vi "IV_Sweep_program1_CEM_Mod2.vi"() -> ()   [LabVIEW 2013]
doc: "I. Description:\nThis example demonstrates how to continuously acquire and generate data at the same time, synchronized with one another.\n\nII. Instructions for Running:\n1. Select the physical channel to correspond to where your signal is input on the DAQ device. Also, select the corresponding channel for where your signal is being generated.\n2. Enter the minimum and maximum voltage ranges.\nNote: For better accuracy try to match the input range to the expected voltage level of the measured signal.\n3. Set the sample rate of the acquisition.\nNote: The rate should be at least twice as fast as the maximum frequency component of the signal being acquired. \n6. Select the Rate for the generation\n7. Select what type of signal to generate and the amplitude.\nNote: This example requires two DMA channels to run. If your hardware does not support two DMA channels, you need to set the Data Transfer Mechanism property for the Analog Output Task to use \"Interrupts\". The Data Transfer Mechanism property is located in the DAQmx Channel Property hierarchy at:\n\nDAQmx Channel Property Node>>Analog Output>>General Properties>>Advanced>>Data Transfer and Memory>>Data Transfer Mechanism\n\nRefer to your device documentation to determine how many DMA channels are supported for your hardware.\n\nIII. Block Diagram Steps:\n1. Create an analog input voltage channel. Also, create an analog output voltage channel.\n2. Set the rate for the sample clock. Additionally, define the sample mode to be continuous. Also, set the sample clock rate for the signal generation.\n2a. Call the Get Terminal Name with Device Prefix VI. This will take a Task and a terminal and create a properly formatted device + terminal name to use as the source of the Trigger.\n3. Define the parameters for a Digital Edge Start Trigger. Set the Analog output to trigger off the AI Start Trigger. This is an internal trigger signal.\n4. Use the Basic Function Generator VI to create the signal to be generated.\n5. Call the Start VI to arm the two functions. Make sure the analog output is armed before the analog input. This will ensure both will start at the same time.\n6. Read the waveform data in a loop until the user hits the stop button or an error occurs. The Is Task Done? VI is used to check for errors in the Analog Output Task.\n7. Call the Clear VI to Clear the Task\n8. Use the popup dialog box to display an error if any.\n\nIV. I/O Connections Overview:\nMake sure your signal input/output terminals match the Physical Channel I/O controls."
uses:
  <vilib>/Utility/error.llb/DialogType.ctl
  <vilib>/DAQmx/read.llb/DAQmx Read (Analog 1D DBL NChan 1Samp).vi
  <vilib>/DAQmx/write.llb/DAQmx Write (Analog DBL 1Chan 1Samp).vi
  <vilib>/DAQmx/create/channels.llb/DAQmx Create Channel (AO-Voltage-Basic).vi
  <vilib>/DAQmx/create/channels.llb/DAQmx Create Channel (AI-Voltage-Basic).vi
  <vilib>/DAQmx/configure/timing.llb/DAQmx Timing (Sample Clock).vi
  <vilib>/DAQmx/miscellaneous.llb/DAQmx Fill In Error Info.vi
  <vilib>/Utility/file.llb/Write To Spreadsheet File (DBL).vi
  <vilib>/Utility/file.llb/Write To Spreadsheet File (I64).vi
panel:
  out "Numeric":i32
  out "x/y":dbl
  in  "Sweep Amplitude":dbl=1.0
  in  "Stop Sweep":bool
  out "Connections 2":string="AI0=Current\nAI1=Bias\nAI2=dI/dV\nAI3=d2I/dV2\nAI4=X-Axis\nAI5=Z-Axis\n"
  out "Connections":string="AO0=Bias\nAO1=Z-axis\nAO2=X-Axis\nAO3=NA"
  in  "Columns":string
  out "Save Indicator":bool
  in  "Update Bias":bool
  in  "Save IV":bool
  in  "Save Decay":bool
  in  "Sweep Bias":bool
  in  "Step Z":bool
  in  "Comment":string="Molecule=C8\nGain=10nA\nBias Gain=div/1\nSweep Freq.=0.005Hz\nRef. Bias=5mV\nRef. Freq=4.33kHz\nGain LIA1=0.5mV\nTC LIA1=300ms\nGain LIA2=\nTC LIA2=\nLIA1=EGG"
  in  "Number Recorded":i32
  in  "DATA Filename":string="Data_"
  in  "Data Directory":path=path "E:/Research/Data"
  out "d2I/dV2":cluster{dbl[], dbl[]}(graph)
  out "dI/dV":cluster{dbl[], dbl[]}(graph)
  out "IV":cluster{dbl[], dbl[]}(graph)
  in  "# Samples":i32=2000
  in  "Frequency (Hz)":dbl=1.0
  in  "stop 3":bool
  in  "Bias":dbl caption="Bias Start Point" step=0.1 format="%_3g"
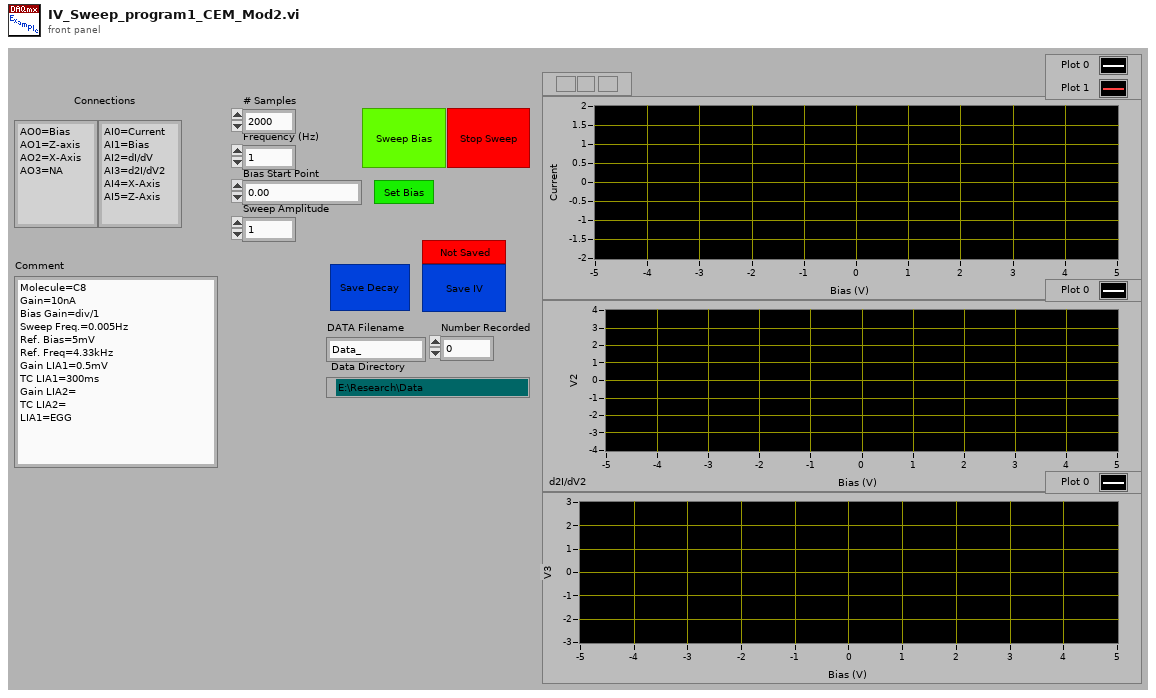
[diagram p1: front panel]
types:
  T1 = enum16{"open", "replace", "create", "open or create", "replace or create", "replace or create with confirmation"}
  T2 = typedef "DialogType.ctl" = u16
  T3 = cluster{dbl[], dbl[], dbl[], dbl[], dbl[], dbl[], dbl[]}
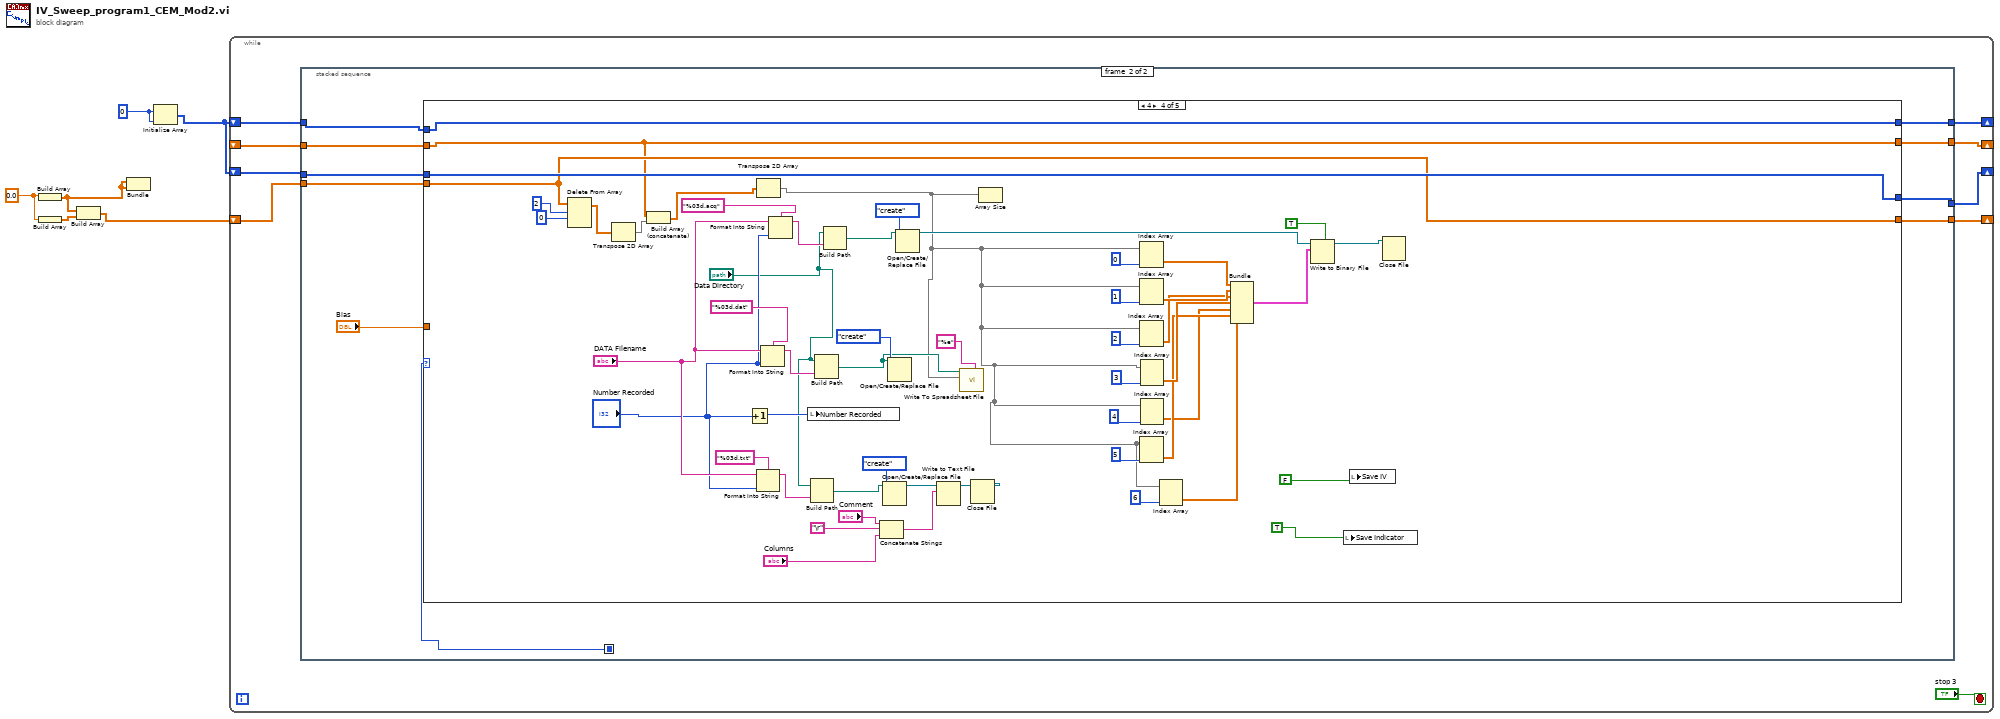
[diagram p0: block diagram]
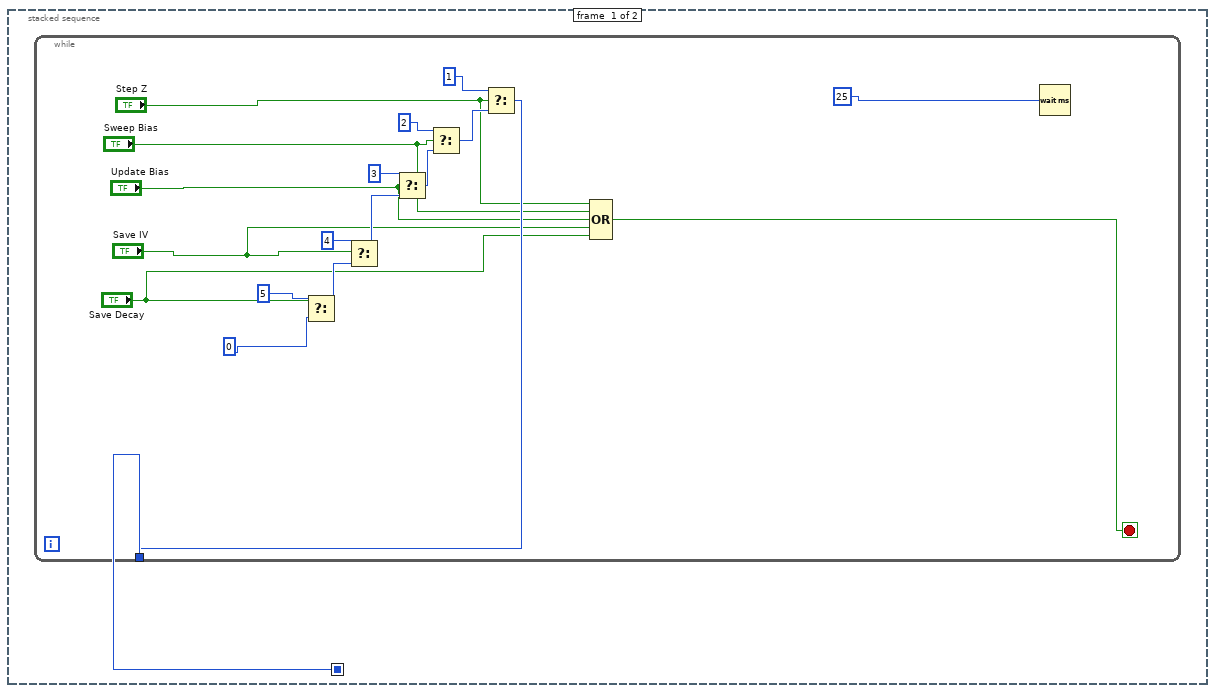
[diagram p2: hidden frame]
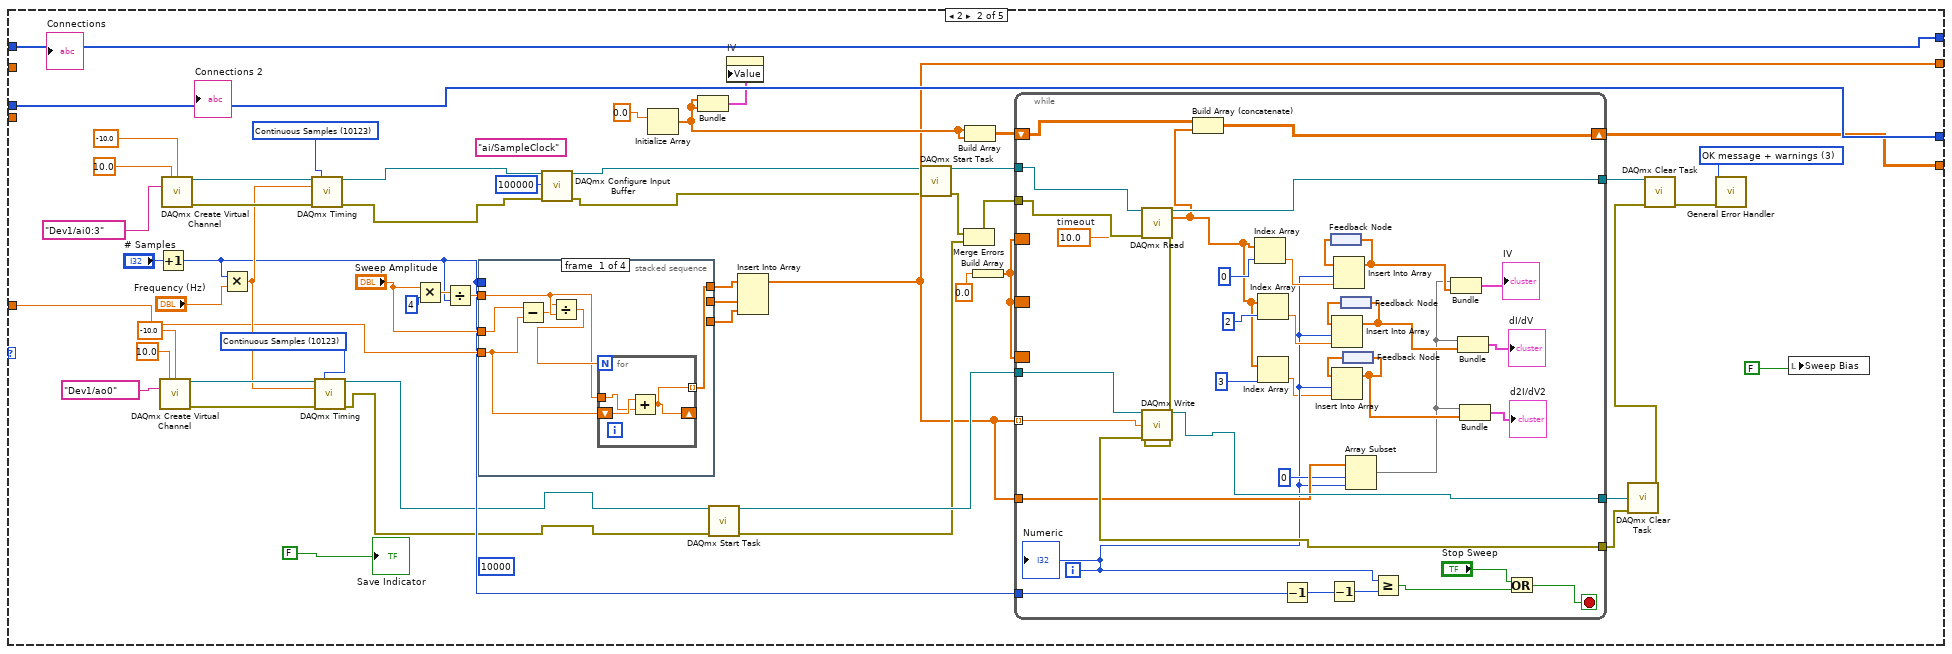
[diagram p4: hidden frame]
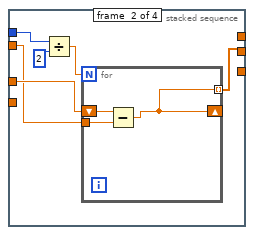
[diagram p5: hidden frame]
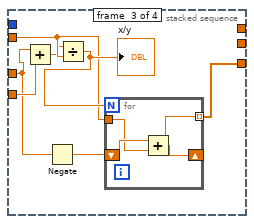
[diagram p6: hidden frame]
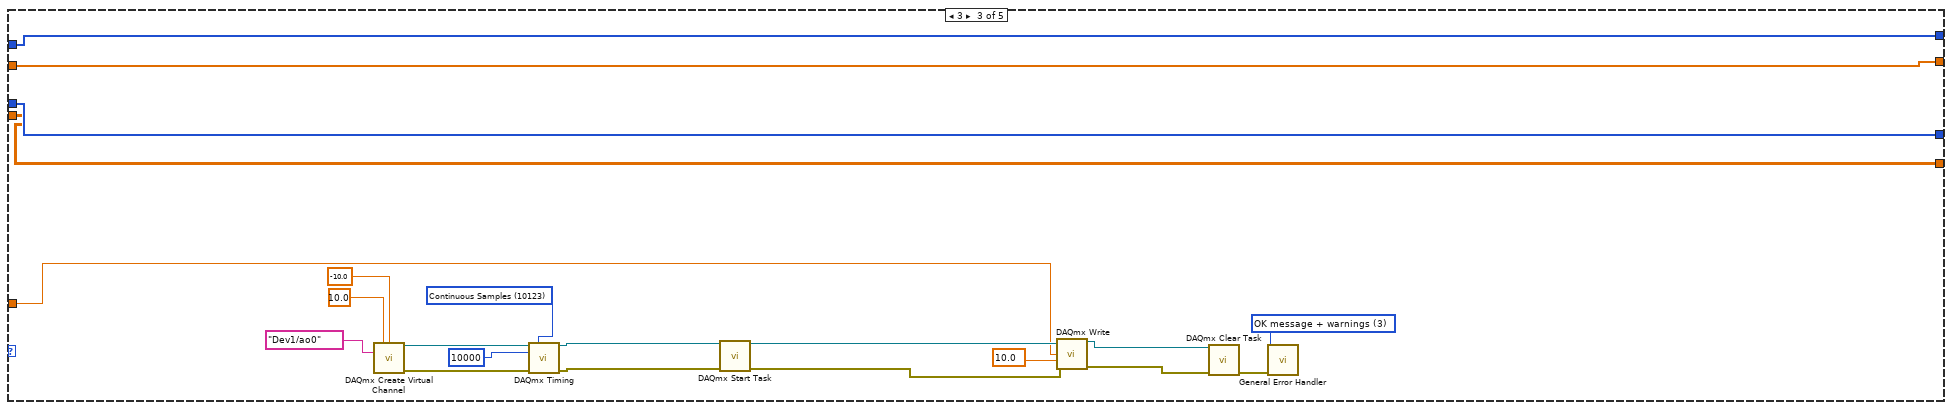
[diagram p8: hidden frame]
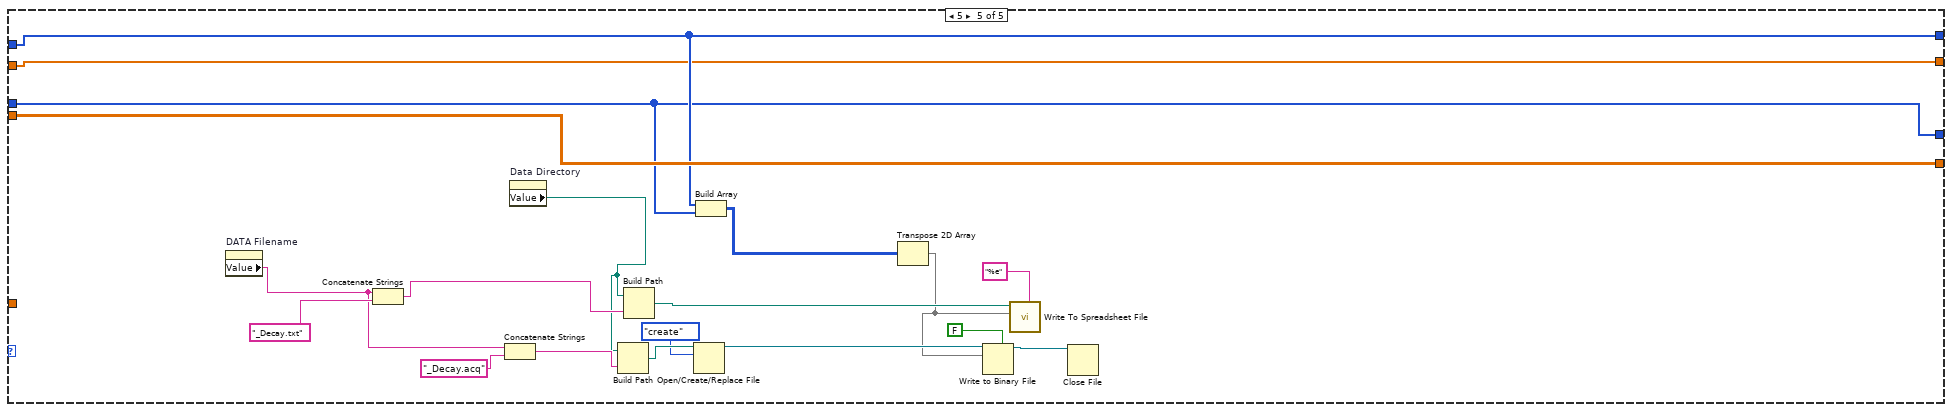
[diagram p9: hidden frame]
diagram:
  w2 = 0
  w6 = 0.0
  n1 = Build Array(w6) -> (w3:dbl[])
  n2 = Build Array(w6) -> (w5:dbl[])
  n3 = Build Array(w3, w5) -> (w4:dbl[][])
  n4 = Bundle(w3, w3) -> ()  [unwired: 1 in, 1 out]
  n5 = Initialize Array(w2, w2) -> (w1:i32[])
  n6 = while {
    shift-right: [w13] -> _
    shift-left: w1 -> [w14]
    shift-right: [w11] -> _
    shift-left: w1 -> [w12]
    shift-right: [w9] -> _
    shift-left: w4 -> [w10]
    shift-right: [w7] -> _
    shift-left: _ -> [w8]
    stop <- "stop 3" stop-if-true
    n7 = stacked-sequence {
      seq-local: [w16 _] -> [_ w44]
      tunnel: w14 -> [_ w43]
      tunnel: [_ w42] -> w13
      tunnel: w12 -> [_ w40]
      tunnel: [_ w39] -> w11
      tunnel: w10 -> [_ w38]
      tunnel: [_ w37] -> w9
      tunnel: w8 -> [_ w36]
      tunnel: [_ w35] -> w7
      frame #0 {
        n8 = while {
          tunnel: [w25] -> w16
          stop <- w24 stop-if-true
          n9 = Select(t=5, s="Save Decay", f=0) -> (s? t:f=w30:i32)
          n10 = Select(t=4, s="Save IV", f=w30) -> (s? t:f=w29:i32)
          n11 = Select(t=3, s="Update Bias", f=w29) -> (s? t:f=w27:i32)
          n12 = Select(t=2, s="Sweep Bias", f=w27) -> (s? t:f=w34:i32)
          n13 = Select(t=1, s="Step Z", f=w34) -> (s? t:f=w25:i32)
          n14 = Compound Arithmetic op=OR("Step Z", "Sweep Bias", "Update Bias", "Save IV", "Save Decay") -> (w24:bool)
          n15 = Wait (ms)(milliseconds to wait=25) -> ()  [unwired: 1 out]
        }
      }
      frame #1 {
        n16 = case shown="4" w44 {
          tunnel: w43 -> [w48 w86 w171 w236 w257]
          tunnel: [w48 w86 w171 w236 w257] -> w42
          tunnel: "Bias" -> [_ w72 w177 _ _]
          tunnel: w40 -> [w47 w83 w172 w237 w258]
          tunnel: [w47 w83 w172 w237 w258] -> w39
          tunnel: w38 -> [w46 _ w169 w216 w259]
          tunnel: [w46 w64 w169 w216 w259] -> w37
          tunnel: [w45 w56 w168 w214 w242] -> w35
          tunnel: w36 -> [w45 _ w168 w214 w242]
          frame 0, Default {
          }
          frame 2 {
            (unwired) 10000
            w81 = 10123 items=["Finite Samples"=10178, "Continuous Samples"=10123, "Hardware Timed Single Point"=12522] ("sample mode")
            w82 = 10123 items=["Finite Samples"=10178, "Continuous Samples"=10123, "Hardware Timed Single Point"=12522] ("sample mode")
            (unwired) "ai/SampleClock" ("terminal")
            w91 = T2 3 items=["no dialog", "OK message", "continue or stop message", "OK message + warnings", "continue/stop + warnings"] ("type of dialog (OK msg:1)")
            n17 = Increment(x="# Samples") -> (x+1=w62:i32)
            n18 = call-poly <vilib>:"DAQmx Create Virtual Channel.vi"("maximum value"=10.0, "minimum value"=-10.0, "physical channels"=tag "Dev1/ao0") -> ("task out"=w94:refnum<k21>, "error out"=w93:errorcluster)  [unwired: 11 in]
            n19 = call-poly <vilib>:"DAQmx Create Virtual Channel.vi"("maximum value"=10.0 ("Maximum Value"), "minimum value"=-10.0 ("Minimum Value"), "physical channels"=tag "Dev1/ai0:3" ("Physical Channel")) -> ("task out"=w98:refnum<k21>, "error out"=w99:errorcluster)  [unwired: 11 in]
            n20 = Multiply(x=w62, y="Frequency (Hz)") -> (x*y=w85:dbl)
            n21 = call-poly <vilib>:"DAQmx Timing.vi"("task/channels in"=w98, "sample mode"=w81, "rate"=w85, "error in"=w99) -> ("task out"=w50:refnum<k21>, "error out"=w52:errorcluster)  [unwired: 10 in]
            n22 = call-poly <vilib>:"DAQmx Timing.vi"("task/channels in"=w94, "sample mode"=w82, "rate"=w85, "error in"=w93) -> ("task out"=w54:refnum<k21>, "error out"=w53:errorcluster)  [unwired: 10 in]
            n23 = Multiply(x="Sweep Amplitude", y=4) -> (x*y=w70:dbl)
            n24 = Divide(x=w70, y=w62) -> (x/y=w69:dbl)
            n25 = stacked-sequence {
              tunnel: "Sweep Amplitude" -> [w145 w151 w159 _]
              tunnel: w72 -> [w143 _ w163 _]
              tunnel: w69 -> [w141 w150 w161 _]
              tunnel: [w142 _ _ _] -> w68
              tunnel: w62 -> [_ w154 _ _]
              tunnel: [_ w149 _ _] -> w67
              tunnel: [_ _ w162 _] -> w66
              frame #0 {
                n26 = Subtract(x=w145, y=w143) -> (x-y=w140:dbl)
                n27 = Divide(x=w140, y=w141) -> (x/y=w144:dbl)
                n28 = for {
                  N: w144 -> [_]
                  tunnel: w141 -> [w147]
                  shift-right: [w146] -> _
                  shift-left: w143 -> [w148]
                  tunnel: [w146] -> w142 mode=indexing
                  n29 = Add(x=w148, y=w147) -> (x+y=w146:dbl)
                }
              }
              frame #1 {
                n30 = Divide(x=w154, y=2) -> (x/y=w152:dbl)
                n31 = for {
                  N: w152 -> [_]
                  tunnel: w150 -> [w156]
                  shift-right: [w155] -> _
                  shift-left: w151 -> [w157]
                  tunnel: [w155] -> w149 mode=indexing
                  n32 = Subtract(x=w157, y=w156) -> (x-y=w155:dbl)
                }
              }
              frame #2 {
                n33 = Add(x=w159, y=w163) -> (x+y=w160:dbl)
                n34 = Negate(x=w159) -> (-x=w158:dbl)
                n35 = Divide(x=w160, y=w161) -> (x/y=w164:dbl)
                "x/y" <- w164
                n36 = for {
                  N: w164 -> [_]
                  tunnel: w161 -> [w166]
                  shift-right: [w165] -> _
                  shift-left: w158 -> [w167]
                  tunnel: [w165] -> w162 mode=indexing
                  n37 = Add(x=w167, y=w166) -> (x+y=w165:dbl)
                }
              }
              frame #3 {
              }
            }
            n38 = call <vilib>:"DAQmx Configure Input Buffer.vi"("task/channels in"=w50, "buffer size (in samples per channel)"=100000, "error in"=w52) -> ("task out"=w49:refnum<k21>, "error out"=w51:errorcluster)  [unwired: 11 in]
            n39 = Initialize Array(0.0) -> (w61:dbl[])  [unwired: 1 in]
            n40 = Bundle(w61, w61) -> (w60:cluster{dbl[], dbl[]})  [unwired: 1 in]
            n41 = call <vilib>:"DAQmx Start Task.vi"("task/channels in"=w54, "error in"=w53) -> ("task out"=w80:refnum<k21>, "error out"=w76:errorcluster)  [unwired: 12 in]
            n42 = property on="IV" class="XYGraph (strict)"("Value"=w60) -> ()  [unwired: 2 in, 2 out]
            n43 = Insert Into Array(array=w68, new element #1=w67, new element #2=w66) -> (w56:dbl[])  [unwired: 1 in]
            n44 = call <vilib>:"DAQmx Start Task.vi"("task/channels in"=w49, "error in"=w51) -> ("task out"=w78:refnum<k21>, "error out"=w77:errorcluster)  [unwired: 12 in]
            n45 = Merge Errors(w77, w76) -> (w79:errorcluster)
            n46 = Build Array(w61, w61) -> (w63:dbl[][])
            n47 = Build Array(0.0) -> (w58:dbl[])
            n48 = while {
              tunnel: [w131] -> w100
              tunnel: [w134] -> w92
              tunnel: [w133] -> w89
              tunnel: w62 -> [w107]
              tunnel: w56 -> [w112] mode=indexing
              tunnel: w80 -> [w136]
              tunnel: w78 -> [w139]
              tunnel: w79 -> [w138]
              shift-right: [w113] -> w64
              shift-left: w63 -> [w132]
              tunnel: w56 -> [w129]
              border: w58 -> [_]
              border: w58 -> [_]
              border: w58 -> [_]
              i -> [w108]
              stop <- w109 stop-if-true
              w135 = 10.0  # timeout
              n49 = call-poly <vilib>:"DAQmx Read.vi"("task/channels in"=w139, "timeout"=w135, "error in"=w138) -> ("task out"=w131:refnum<k21>, "data"=w103:dbl[], "error out"=w137:errorcluster)  [unwired: 10 in]
              n50 = call-poly <vilib>:"DAQmx Write.vi"("task/channels in"=w136, "data"=w112, "error in"=w137) -> ("task out"=w134:refnum<k21>, "error out"=w133:errorcluster)  [unwired: 10 in, 1 out]
              n51 = Build Array (concatenate)(w132, w103) -> (w113:dbl[][])
              n52 = Index Array(array=w103, index=0) -> (element=w126:dbl)
              n53 = Index Array(array=w103, index=2) -> (element=w122:dbl)
              n54 = Index Array(array=w103, index=3) -> (element=w104:dbl)
              n55 = Decrement(x=w107) -> (x-1=w105:i32)
              n56 = Decrement(x=w105) -> (x-1=w106:i32)
              n57 = feedback #1() -> (w125:dbl[])
              n58 = Insert Into Array(array=w125, index=w108, new element=w126) -> (w127:dbl[])
              n59 = feedback-in #1(w127) -> ()
              n60 = feedback #2() -> (w121:dbl[])
              n61 = Insert Into Array(array=w121, index=w108, new element=w122) -> (w119:dbl[])
              n62 = feedback-in #2(w119) -> ()
              n63 = feedback #3() -> (w120:dbl[])
              n64 = Insert Into Array(array=w120, index=w108, new element=w104) -> (w118:dbl[])
              n65 = feedback-in #3(w118) -> ()
              n66 = Array Subset(array=w129, index=0, length=w108) -> (w117:dbl[])
              n67 = Greater Or Equal?(x=w108, y=w106) -> (x >= y?=w110:bool)
              n68 = Bundle(w117, w127) -> (→"IV":cluster{dbl[], dbl[]})  [unwired: 1 in]
              n69 = Bundle(w117, w119) -> (→"dI/dV":cluster{dbl[], dbl[]})  [unwired: 1 in]
              n70 = Bundle(w117, w118) -> (→"d2I/dV2":cluster{dbl[], dbl[]})  [unwired: 1 in]
              n71 = Or(x="Stop Sweep", y=w110) -> (x .or. y?=w109:bool)
              "Numeric" <- w108
            }
            n72 = call <vilib>:"DAQmx Clear Task.vi"("task in"=w92, "error in"=w89) -> ("error out"=w88:errorcluster)  [unwired: 13 in]
            n73 = call <vilib>:"DAQmx Clear Task.vi"("task in"=w100, "error in"=w88) -> ("error out"=w87:errorcluster)  [unwired: 13 in]
            n74 = call <vilib>:"General Error Handler.vi"("type of dialog (OK msg:1)"=w91, "error in (no error)"=w87) -> ()  [unwired: 9 in, 5 out]
            n75 = local write "Sweep Bias"(FALSE) -> ()
            "Save Indicator" <- FALSE
          }
          frame 3 {
            w176 = T2 3 items=["no dialog", "OK message", "continue or stop message", "OK message + warnings", "continue/stop + warnings"] ("type of dialog (OK msg:1)")
            w182 = 10123 items=["Finite Samples"=10178, "Continuous Samples"=10123, "Hardware Timed Single Point"=12522] ("sample mode")
            n76 = call-poly <vilib>:"DAQmx Create Virtual Channel.vi"("maximum value"=10.0 ("maximum value 2"), "minimum value"=-10.0 ("minimum value 2"), "physical channels"=tag "Dev1/ao0" ("physical channels 2")) -> ("task out"=w185:refnum<k21>, "error out"=w184:errorcluster)  [unwired: 11 in]
            n77 = call-poly <vilib>:"DAQmx Timing.vi"("task/channels in"=w185, "sample mode"=w182, "rate"=10000, "error in"=w184) -> ("task out"=w181:refnum<k21>, "error out"=w180:errorcluster)  [unwired: 10 in]
            n78 = call <vilib>:"DAQmx Start Task.vi"("task/channels in"=w181, "error in"=w180) -> ("task out"=w179:refnum<k21>, "error out"=w178:errorcluster)  [unwired: 12 in]
            n79 = call-poly <vilib>:"DAQmx Write.vi"("task/channels in"=w179, "data"=w177, "timeout"=10.0 ("Wirite Timeout"), "error in"=w178) -> ("task out"=w174:refnum<k21>, "error out"=w173:errorcluster)  [unwired: 9 in, 1 out]
            n80 = call <vilib>:"DAQmx Clear Task.vi"("task in"=w174, "error in"=w173) -> ("error out"=w175:errorcluster)  [unwired: 13 in]
            n81 = call <vilib>:"General Error Handler.vi"("type of dialog (OK msg:1)"=w176, "error in (no error)"=w175) -> ()  [unwired: 9 in, 5 out]
          }
          frame 4 {
            n82 = Delete From Array(array=w216, length=2, index (row)=0) -> (array with subset deleted=w213:dbl[][])  [unwired: 1 in, 1 out]
            n83 = Transpose 2D Array(2D array=w213) -> (transposed array=w212:dbl[][])
            n84 = Build Array (concatenate)(w214, w212) -> (w211:dbl[][])
            n85 = Increment(x="Number Recorded") -> (x+1=w239:i32)
            n86 = Format Into String(format string="%03d.txt", initial string="DATA Filename", "Number Recorded") -> (resulting string=w227:string)  [unwired: 1 in, 1 out]
            n87 = Transpose 2D Array(2D array=w211) -> (transposed array=w198:dbl[][])
            n88 = Format Into String(format string="%03d.dat", initial string="DATA Filename", "Number Recorded") -> (resulting string=w241:string)  [unwired: 1 in, 1 out]
            n89 = Format Into String(format string="%03d.acq", initial string="DATA Filename", "Number Recorded") -> (resulting string=w234:string)  [unwired: 1 in, 1 out]
            n90 = local write "Number Recorded"(w239) -> ()
            n91 = Build Path(base path="Data Directory", name or relative path=w227) -> (appended path=w225:path)
            n92 = Build Path(base path="Data Directory", name or relative path=w241) -> (appended path=w238:path)
            n93 = Build Path(base path="Data Directory", name or relative path=w234) -> (appended path=w232:path)
            n94 = Concatenate Strings("Comment", "\r", "Columns") -> (w208:string)
            n95 = Open/Create/Replace File(file path (use dialog)=w225, operation (0:open)=T1."create") -> (refnum out=w220:refnum<file>)  [unwired: 4 in, 2 out]
            n96 = Open/Create/Replace File(file path (use dialog)=w238, operation (0:open)=T1."create") -> ()  [unwired: 4 in, 3 out]
            n97 = Open/Create/Replace File(file path (use dialog)=w232, operation (0:open)=T1."create") -> (refnum out=w231:refnum<file>)  [unwired: 4 in, 2 out]
            n98 = Write to Text File(file (use dialog)=w220, text=w208) -> (refnum out=w219:refnum<file>)  [unwired: 2 in, 2 out]
            n99 = call-poly <vilib>:"Write To Spreadsheet File.vi"("format (%.3f)"="%e", "2D data"=w198, "file path (dialog if empty)"=w238) -> ()  [unwired: 5 in, 1 out]
            n100 = Close File(refnum=w219) -> ()  [unwired: 1 in, 2 out]
            n101 = Array Size(array=w198) -> ()  [unwired: 1 out]
            n102 = Index Array(array=w198, index (col)=0) -> (element=w197:dbl[])  [unwired: 1 in]
            n103 = Index Array(array=w198, index (col)=1) -> (element=w196:dbl[])  [unwired: 1 in]
            n104 = Index Array(array=w198, index (col)=2) -> (element=w195:dbl[])  [unwired: 1 in]
            n105 = Index Array(array=w198, index (col)=5) -> (element=w193:dbl[])  [unwired: 1 in]
            n106 = Index Array(array=w198, index (col)=3) -> (element=w194:dbl[])  [unwired: 1 in]
            n107 = Index Array(array=w198, index (col)=4) -> (element=w189:dbl[])  [unwired: 1 in]
            n108 = Index Array(array=w198, index (col)=6) -> (element=w192:dbl[])  [unwired: 1 in]
            n109 = Bundle(w197, w196, w195, w194, w189, w193, w192) -> (w191:T3)  [unwired: 1 in]
            n110 = Write to Binary File(file (use dialog)=w231, data=w191, 5:TRUE ("prepend array or string size? (T)")) -> (refnum out=w229:refnum<file>)  [unwired: 3 in, 2 out]
            n111 = local write "Save Indicator"(TRUE) -> ()
            n112 = local write "Save IV"(FALSE) -> ()
            n113 = Close File(refnum=w229) -> ()  [unwired: 1 in, 2 out]
          }
          frame 5 {
            n114 = property on="DATA Filename" class="Str"() -> ("Value"=w252:string)  [unwired: 2 in, 2 out]
            n115 = Concatenate Strings(w252, "_Decay.txt") -> (w256:string)
            n116 = Concatenate Strings(w252, "_Decay.acq") -> (w250:string)
            n117 = property on="Data Directory" class="Path"() -> ("Value"=w249:path)  [unwired: 2 in, 2 out]
            n118 = Build Path(base path=w249, name or relative path=w250) -> (appended path=w248:path)
            n119 = Build Path(base path=w249, name or relative path=w256) -> (appended path=w255:path)
            n120 = Open/Create/Replace File(file path (use dialog)=w248, operation (0:open)=T1."create") -> (refnum out=w254:refnum<file>)  [unwired: 4 in, 2 out]
            n121 = Build Array(w258, w257) -> (w245:i32[][])
            n122 = Transpose 2D Array(2D array=w245) -> (transposed array=w244:i32[][])
            n123 = Write to Binary File(file (use dialog)=w254, data=w244, 5:FALSE ("prepend array or string size? (T)")) -> (refnum out=w253:refnum<file>)  [unwired: 3 in, 2 out]
            n124 = call-poly <vilib>:"Write To Spreadsheet File.vi"("format (%d)"="%e", "2D data"=w244, "file path (dialog if empty)"=w255) -> ()  [unwired: 5 in, 1 out]
            n125 = Close File(refnum=w253) -> ()  [unwired: 1 in, 2 out]
          }
        }
      }
    }
  }
